vi "HTTPMethod.vi"(4 "HttpRequestMessage":refnum<class "HttpRequestMessage.lvclass">, 6 "Timeout_ms (10000)":i32=10000, 7 "Method":T1, 8 "error in (no error)":errorcluster, 9 "HttpContent":refnum<class "HttpContent.lvclass">, 10 "URL":string, 11 "LabVIEWHTTPClient_NET in":refnum<class "LabVIEWHTTPClient_NET.lvclass">) -> (0 "error out":errorcluster, 2 "HttpResponseMessage out":refnum<class "HttpResponseMessage.lvclass">, 3 "LabVIEWHTTPClient_NET out":refnum<class "LabVIEWHTTPClient_NET.lvclass">)   [LabVIEW 2018, in "LabVIEWHTTPClient_NET.lvlib" / "LabVIEWHTTPClient_NET.lvclass"]
uses:
  LabVIEWHTTPClient_NET.lvclass
  Types/method_enum.ctl
  HttpResponseMessage/HttpResponseMessage.lvclass
  HttpRequestMessage/HttpRequestMessage.lvclass
  HttpContent/HttpContent.lvclass
  HttpContent/HttpContent.lvclass/HttpContent.ctl
  HttpRequestMessage/HttpRequestMessage.lvclass/HttpRequestMessage.ctl
  LabVIEWHTTPClient_NET.lvclass/LabVIEWHTTPClient_NET.ctl
  HttpRequestMessage/Accessors/Read NET_HttpRequestMessage.vi
  HttpContent/Accessors/Read NET_HttpContent.vi
  Accessors/Read NET_HttpClient.vi
  Accessors/Read RequestHeaderContentFirst.vi
  System.Net.Http
  LabVIEWHTTPClient_NET.lvlib
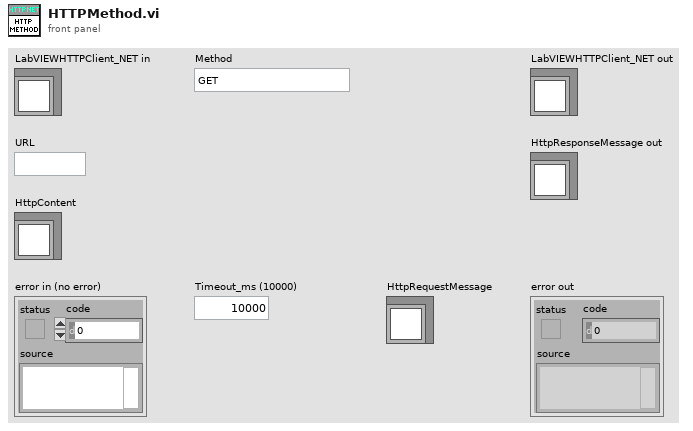
[diagram p1: front panel]
types:
  T1 = typedef "LabVIEWHTTPClient_NET.lvlib/method_enum.ctl" = enum16{"GET", "PUT", "POST", "DELETE", "HEAD", "TRACE", "SEND"}
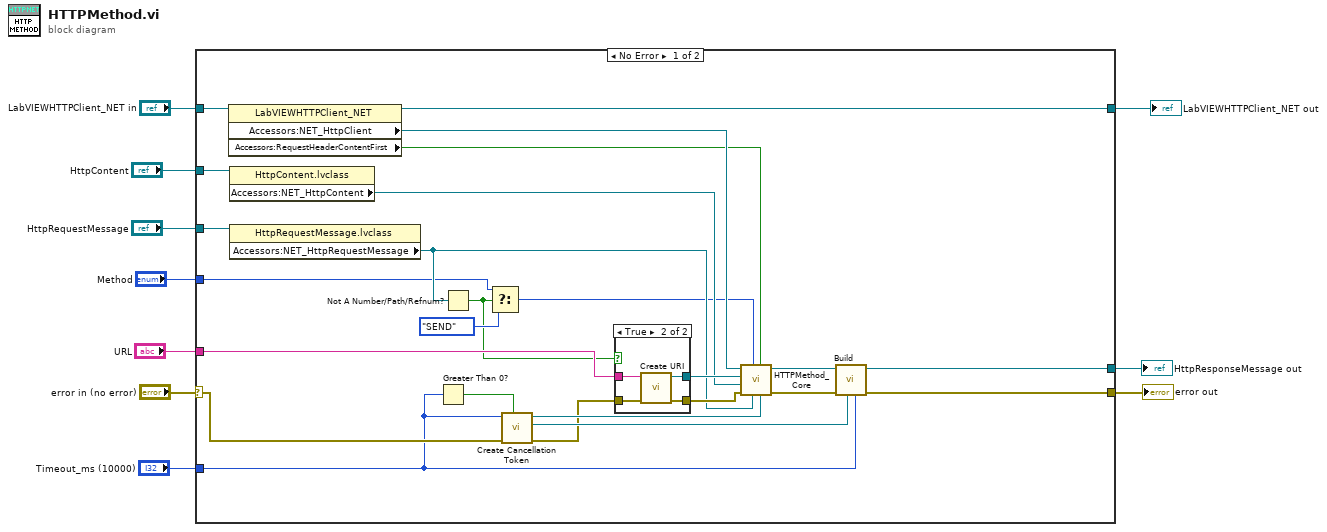
[diagram p0: block diagram]
diagram:
  n1 = case shown="No Error" "error in (no error)" {
    selector: "error in (no error)" -> [w22 w42]
    tunnel: [w27 w42] -> w9
    tunnel: [w34 w41] -> w7
    tunnel: "LabVIEWHTTPClient_NET in" -> [w35 w41]
    tunnel: "Method" -> [w17 _]
    tunnel: "Timeout_ms (10000)" -> [w12 _]
    tunnel: [w25 _] -> w4
    tunnel: "URL" -> [w23 _]
    tunnel: "HttpContent" -> [w21 _]
    tunnel: "HttpRequestMessage" -> [w20 _]
    frame No Error {
      n2 = property class="LabVIEWHTTPClient_NET"(reference=w35) -> (reference out=w34:refnum<class "LabVIEWHTTPClient_NET.lvclass">, "Accessors:NET_HttpClient"=w33:refnum<k24>, "Accessors:RequestHeaderContentFirst"=w13:bool)  [unwired: 1 in, 1 out]
      n3 = property class="HttpContent.lvclass"(reference=w21) -> ("Accessors:NET_HttpContent"=w19:refnum<k24>)  [unwired: 1 in, 2 out]
      n4 = property class="HttpRequestMessage.lvclass"(reference=w20) -> ("Accessors:NET_HttpRequestMessage"=w18:refnum<k24>)  [unwired: 1 in, 2 out]
      n5 = Greater Than 0?(x=w12) -> (x > 0?=w11:bool)
      n6 = Not A Number/Path/Refnum?(number/path/refnum=w18) -> (NaN/Path/Refnum?=w14:bool)
      n7 = Select(t=w17, s=w14, f=method_enum."SEND") -> (s? t:f=w15:T1)
      n8 = call "Create Cancellation Token.vi"("IncludeTimeout (T)"=w11, "error in (no error)"=w22, "Timeout_ms (10000)"=w12) -> ("error out"=w24:errorcluster, "NET_CancellationSource"=w26:refnum<k24>, "NET_CancellationToken"=w29:refnum<k24>)  [unwired: 6 in]
      n9 = case shown="True" w14 {
        tunnel: [_ w40] -> w32
        tunnel: [w36 w39] -> w31
        tunnel: w24 -> [w36 w38]
        tunnel: w23 -> [_ w37]
        frame False {
        }
        frame True {
          n10 = call "Create URI.vi"("error in (no error)"=w38, "uriString"=w37) -> ("error out"=w39:errorcluster, ".NET Refnum out"=w40:refnum<k24>)  [unwired: 8 in]
        }
      }
      n11 = call "HTTPMethod_Core.vi"("cancellationToken"=w29, "ReturnHeadersFirst"=w13, "HttpRequest"=w18, "Method"=w15, "error in (no error)"=w31, "HttpContent"=w19, "uri"=w32, "HttpClient"=w33) -> ("error out"=w28:errorcluster, "HttpResponseMessage"=w30:refnum<k24>)  [unwired: 2 in]
      n12 = call "Build.vi"("Timeout_ms"=w12, "NET_CancellationSource"=w26, "error in (no error)"=w28, "NET_HttpResponseMessage"=w30) -> ("error out"=w27:errorcluster, "HttpResponseMessage out"=w25:refnum<class "HttpResponseMessage.lvclass">)  [unwired: 6 in]
    }
    frame Error {
    }
  }
  "error out" <- w9
  "LabVIEWHTTPClient_NET out" <- w7
  "HttpResponseMessage out" <- w4
